vi "LXI Command String.vi"(10 "LXI Triggers":bool[](array[boolean])=[TRUE, TRUE, TRUE, TRUE, TRUE, TRUE, TRUE, TRUE]) -> (2 "LXI Command String":string)   [LabVIEW 2023, in "Agilent B2900 Series.lvlib"]
doc: "Parse LXI Triggers array which contains 8 booleans to indicate the use of specified LXI Triggers to a comma separated string accepted by SCPI Command"
uses:
  Agilent B2900 Series.lvlib
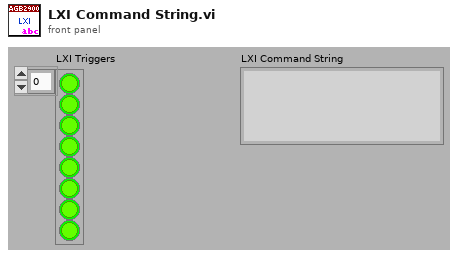
[diagram p1: front panel]
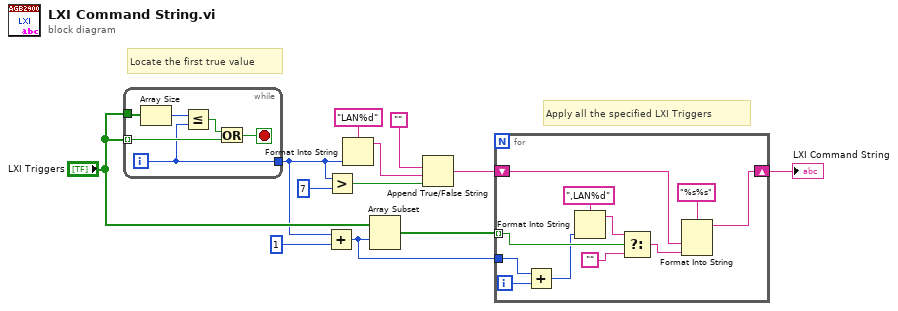
[diagram p0: block diagram]
diagram:
  # "Apply all the specified LXI Triggers"
  # "Locate the first true value"
  n1 = while {
    tunnel: "LXI Triggers" -> [w17] mode=indexing
    tunnel: [w14] -> w6
    tunnel: "LXI Triggers" -> [w18]
    i -> [w14]
    stop <- w16 stop-if-true
    n2 = Array Size(array=w18) -> (size(s)=w15:i32)
    n3 = Less Or Equal?(x=w15, y=w14) -> (x <= y?=w13:bool)
    n4 = Or(x=w13, y=w17) -> (x .or. y?=w16:bool)
  }
  n5 = Add(x=w6, y=1) -> (x+y=w8:i32)
  n6 = Greater?(x=w6, y=7) -> (0:w4:bool)
  n7 = Format Into String(format string="LAN%d", w6) -> (resulting string=w3:string)  [unwired: 2 in, 1 out]
  n8 = Array Subset(array="LXI Triggers", index=w8) -> (w11:bool[])  [unwired: 1 in]
  n9 = Append True/False String(1:w4, 2:w3, 3:"") -> (0:w2:string)  [unwired: 1 in]
  n10 = for {
    shift-right: [w22] -> w9
    shift-left: w2 -> [w20]
    tunnel: w11 -> [w26] mode=indexing
    tunnel: w8 -> [w23]
    i -> [w25]
    n11 = Add(x=w23, y=w25) -> (x+y=w24:i32)
    n12 = Format Into String(format string=",LAN%d", w24) -> (resulting string=w29:string)  [unwired: 2 in, 1 out]
    n13 = Select(t=w29, s=w26, f="") -> (s? t:f=w21:string)
    n14 = Format Into String(format string="%s%s", w20, w21) -> (resulting string=w22:string)  [unwired: 2 in, 1 out]
  }
  "LXI Command String" <- w9
